vi "Graph_show_hide (SubVI).vi"(5 "XYGraph in":refnum<vi>, 7 "Hide/Show":enum16{"Show", "Hide"}(ring), 8 "Error In":errorcluster, 9 "String in":string, 10 "CmbBox Refnum":refnum<vi>, 11 "Arr Refnum":refnum<vi>) -> (0 "Error Out":errorcluster)   [LabVIEW 2018]
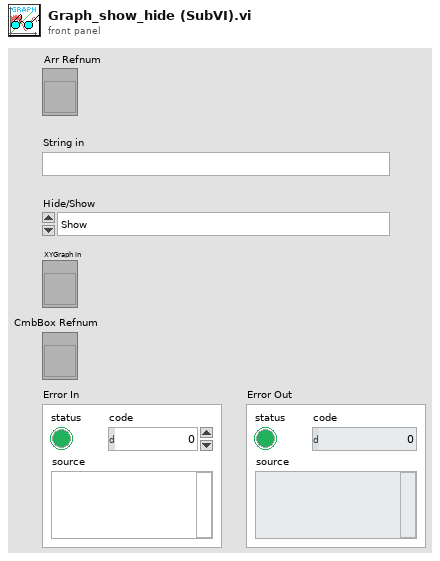
[diagram p1: front panel]
types:
  T1 = typedef "LVComboBoxStrsAndValuesArrayTypeDef.ctl" = cluster{"String":string, "Value":string}[]
  T2 = typedef "Line.ctl" = cluster{"Width":dbl, "Color":i64, "Array Oy":dbl[], "Array Ox":dbl[], "Name":string, "Plot Visible":T3}
  T3 = typedef "View.ctl" = bool
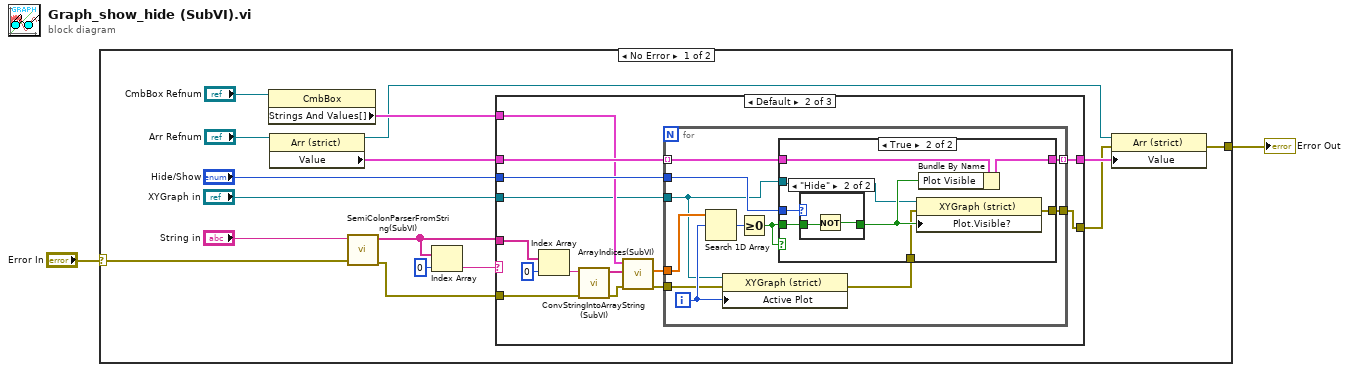
[diagram p0: block diagram]
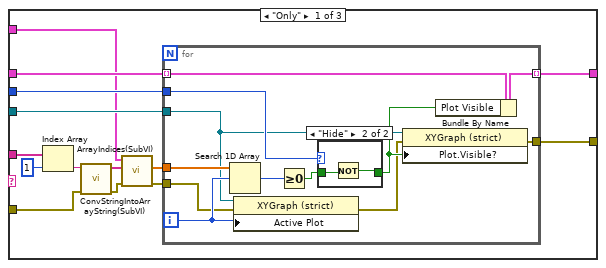
[diagram p2: hidden frame]
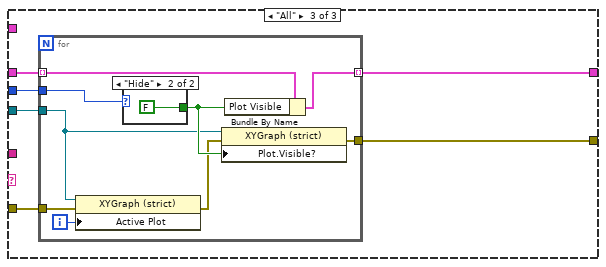
[diagram p6: hidden frame]
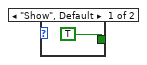
[diagram p7: hidden frame]
diagram:
  n1 = case shown="No Error" "Error In" {
    selector: "Error In" -> [w7 w103]
    tunnel: [w4 w103] -> w1
    frame No Error {
      n2 = property on="Property Node" class="CmbBox"(reference="CmbBox Refnum") -> ("Strings And Values[]"=w12:T1)  [unwired: 1 in, 2 out]
      n3 = property on="Property Node" class="Arr (strict)"(reference="Arr Refnum") -> (reference out=w8:refnum<vi>, "Value"=w10:T2[])  [unwired: 1 in, 1 out]
      n4 = call "SemiColonParserFromString(SubVI).vi"("Error In"=w7, "String In"="String in") -> ("Error Out"=w6:errorcluster, "String Array Out"=w14:string[])  [unwired: 8 in]
      n5 = Index Array(array=w14, index=0) -> (element=w15:string)
      n6 = case shown="Default" w15 {
        tunnel: w14 -> [w30 w59 _]
        tunnel: w10 -> [w29 w58 w91]
        tunnel: [w28 w57 w90] -> w9
        tunnel: "Hide/Show" -> [w27 w56 w89]
        tunnel: "XYGraph in" -> [w26 w52 w88]
        tunnel: w12 -> [w23 w53 _]
        tunnel: w6 -> [w22 w51 w87]
        tunnel: [w19 w48 w86] -> w5
        frame "Only" {
          n7 = Index Array(array=w30, index=1) -> (element=w32:string)
          n8 = call "ConvStringIntoArrayString(SubVI).vi"("Error In"=w22, "String In"=w32) -> ("Error Out"=w21:errorcluster, "Array String Out"=w25:string[])  [unwired: 8 in]
          n9 = call "ArrayIndices(SubVI).vi"("Error In"=w21, "Array In"=w25, "StringsAndValues[]"=w23) -> ("Error Out"=w20:errorcluster, "Array Out"=w24:dbl[])  [unwired: 7 in]
          n10 = for {
            tunnel: w24 -> [w44]
            tunnel: w29 -> [w41] mode=indexing
            tunnel: [w40] -> w28 mode=indexing
            tunnel: w27 -> [w39]
            tunnel: w26 -> [w33]
            tunnel: w20 -> [w35]
            tunnel: [w34] -> w19
            i -> [w42]
            n11 = Search 1D Array(1D array=w44, element=w42) -> (index of element=w43:i32)  [unwired: 1 in]
            n12 = property on="Property Node" class="XYGraph (strict)"(reference=w33, error in=w35, "Active Plot"=w42) -> (error out=w36:errorcluster)  [unwired: 1 out]
            n13 = Greater Or Equal To 0?(x=w43) -> (x >= 0?=w38:bool)
            n14 = case shown="\"Hide\"" w39 {
              tunnel: [w45 w46] -> w37
              tunnel: w38 -> [w45 w47]
              frame "Show", Default {
              }
              frame "Hide" {
                n15 = Not(x=w47) -> (.not. x?=w46:bool)
              }
            }
            n16 = property on="Property Node" class="XYGraph (strict)"(reference=w33, error in=w36, "Plot.Visible?"=w37) -> (error out=w34:errorcluster)  [unwired: 1 out]
            n17 = Bundle By Name(cluster=w41, "Plot Visible"=w37) -> (w40:T2)
          }
        }
        frame Default {
          n18 = Index Array(array=w59, index=0) -> (element=w61:string)
          n19 = call "ConvStringIntoArrayString(SubVI).vi"("Error In"=w51, "String In"=w61) -> ("Error Out"=w50:errorcluster, "Array String Out"=w55:string[])  [unwired: 8 in]
          n20 = call "ArrayIndices(SubVI).vi"("Error In"=w50, "Array In"=w55, "StringsAndValues[]"=w53) -> ("Error Out"=w49:errorcluster, "Array Out"=w54:dbl[])  [unwired: 7 in]
          n21 = for {
            tunnel: w54 -> [w72]
            tunnel: w58 -> [w69] mode=indexing
            tunnel: [w68] -> w57 mode=indexing
            tunnel: w56 -> [w66]
            tunnel: w52 -> [w62]
            tunnel: w49 -> [w65]
            tunnel: [w63] -> w48
            i -> [w70]
            n22 = Search 1D Array(1D array=w72, element=w70) -> (index of element=w71:i32)  [unwired: 1 in]
            n23 = property on="Property Node" class="XYGraph (strict)"(reference=w62, error in=w65, "Active Plot"=w70) -> (error out=w64:errorcluster)  [unwired: 1 out]
            n24 = Greater Or Equal To 0?(x=w71) -> (x >= 0?=w67:bool)
            n25 = case shown="True" w67 {
              tunnel: w69 -> [w74 w82]
              tunnel: [w74 w81] -> w68
              tunnel: w67 -> [_ w79]
              tunnel: w66 -> [_ w78]
              tunnel: w62 -> [_ w77]
              tunnel: w64 -> [w73 w76]
              tunnel: [w73 w75] -> w63
              frame False {
              }
              frame True {
                n26 = case shown="\"Hide\"" w78 {
                  tunnel: [w83 w84] -> w80
                  tunnel: w79 -> [w83 w85]
                  frame "Show", Default {
                  }
                  frame "Hide" {
                    n27 = Not(x=w85) -> (.not. x?=w84:bool)
                  }
                }
                n28 = property on="Property Node" class="XYGraph (strict)"(reference=w77, error in=w76, "Plot.Visible?"=w80) -> (error out=w75:errorcluster)  [unwired: 1 out]
                n29 = Bundle By Name(cluster=w82, "Plot Visible"=w80) -> (w81:T2)
              }
            }
          }
        }
        frame "All" {
          n30 = for {
            tunnel: w91 -> [w100] mode=indexing
            tunnel: [w99] -> w90 mode=indexing
            tunnel: w89 -> [w97]
            tunnel: w88 -> [w92]
            tunnel: w87 -> [w94]
            tunnel: [w93] -> w86
            i -> [w98]
            n31 = property on="Property Node" class="XYGraph (strict)"(reference=w92, error in=w94, "Active Plot"=w98) -> (error out=w95:errorcluster)  [unwired: 1 out]
            n32 = case shown="\"Hide\"" w97 {
              tunnel: [TRUE FALSE] -> w96
              frame "Show", Default {
              }
              frame "Hide" {
              }
            }
            n33 = property on="Property Node" class="XYGraph (strict)"(reference=w92, error in=w95, "Plot.Visible?"=w96) -> (error out=w93:errorcluster)  [unwired: 1 out]
            n34 = Bundle By Name(cluster=w100, "Plot Visible"=w96) -> (w99:T2)
          }
        }
      }
      n35 = property on="Property Node" class="Arr (strict)"(reference=w8, error in=w5, "Value"=w9) -> (error out=w4:errorcluster)  [unwired: 1 out]
    }
    frame Error {
    }
  }
  "Error Out" <- w1
